vi "ex5_list_cameras.vi"() -> ()   [LabVIEW 2012]
panel:
  out "error out":errorcluster
  in  "error in (no error)":errorcluster
  out "Number of Cameras":u32
  out "ID 4":u32
  out "Cam 4":bool
  out "ID 3":u32
  out "Cam 3":bool
  out "ID 2":u32
  out "Cam 2":bool
  out "ID 1":u32
  out "Cam 1":bool
  # "Unique IDs of the first four cameras available"
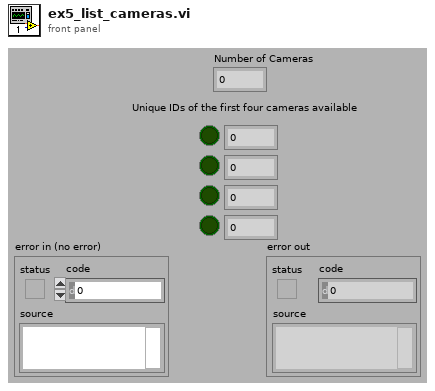
[diagram p1: front panel]
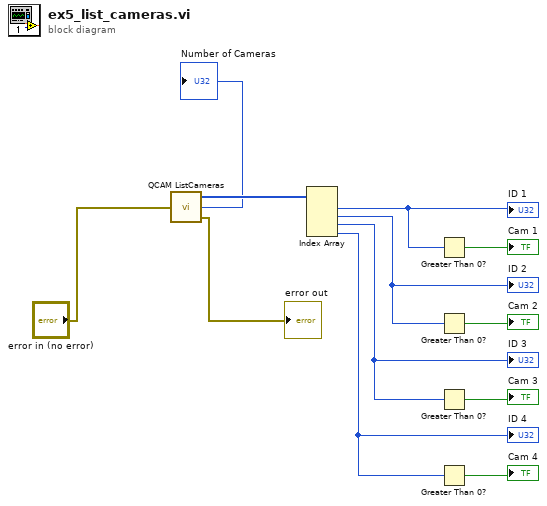
[diagram p0: block diagram]
diagram:
  n1 = call <userlib>:"QCAM ListCameras.vi"("error in (no error)"="error in (no error)") -> ("Unique IDs"=w8:u32[], "Number of cameras"=→"Number of Cameras":u32, "error out"=→"error out":errorcluster)
  n2 = Index Array(array=w8) -> (element #1=w7:u32, element #2=w6:u32, element #3=w5:u32, element #4=w4:u32)  [unwired: 4 in]
  "ID 1" <- w7
  "ID 2" <- w6
  "ID 3" <- w5
  "ID 4" <- w4
  n3 = Greater Than 0?(x=w7) -> (x > 0?=→"Cam 1":bool)
  n4 = Greater Than 0?(x=w6) -> (x > 0?=→"Cam 2":bool)
  n5 = Greater Than 0?(x=w5) -> (x > 0?=→"Cam 3":bool)
  n6 = Greater Than 0?(x=w4) -> (x > 0?=→"Cam 4":bool)
